vi "Get Transceiver Count.vi"(11 "Framework in":refnum<class "Framework.lvclass">) -> (2 "transceiver count":i32, 3 "Framework out":refnum<class "Framework.lvclass">)   [LabVIEW 2017, in "Data Sharing Framework Core.lvlib" / "Data Sharing Framework Engine.lvlib" / "Framework.lvclass"]
uses:
  Framework.lvclass
  Framework.lvclass/Framework.ctl
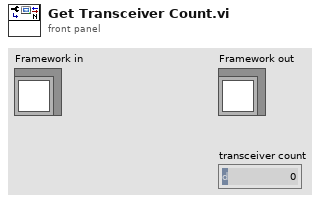
[diagram p1: front panel]
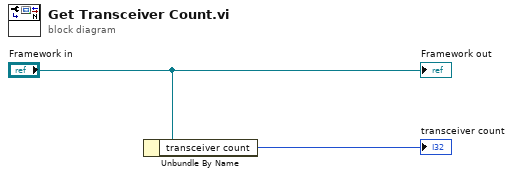
[diagram p0: block diagram]
diagram:
  n1 = Unbundle By Name("Framework in") -> ("transceiver count"=→"transceiver count":i32)
  "Framework out" <- "Framework in"
